vi "Manage Memory.vi"(8 "error in (no error)":errorcluster, 9 "User Waveform (0)":i32, 10 "Memory Operation (0: List Memory)":i32(ring) items=["List Memory", "Copy to User Waveform", "Copy from User Waveform"], 11 "VISA resource name":refnum<visa-resource-name>) -> (0 "error out":errorcluster, 2 "Memory List":string, 3 "VISA resource name out":refnum<visa-resource-name>)   [LabVIEW 2016, in "Tektronix AFG 1000 Series.lvlib"]
doc: "Copy or list memory waveforms."
uses:
  Tektronix AFG 1000 Series.lvlib
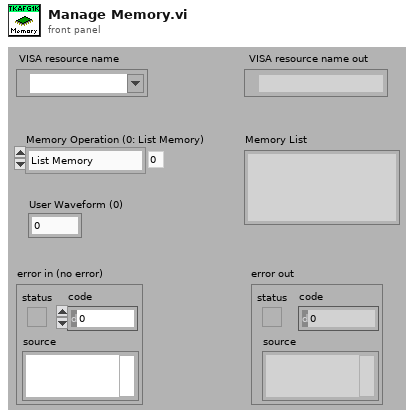
[diagram p1: front panel]
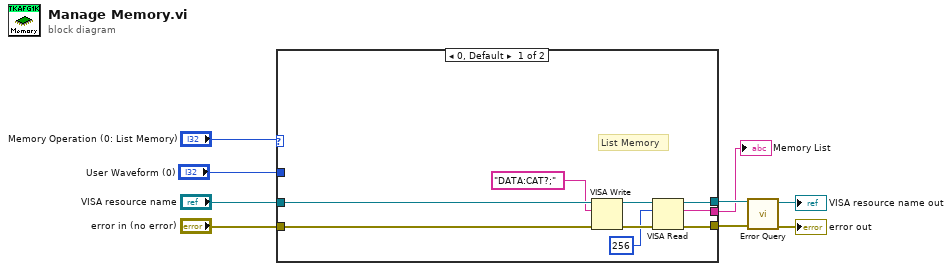
[diagram p0: block diagram]
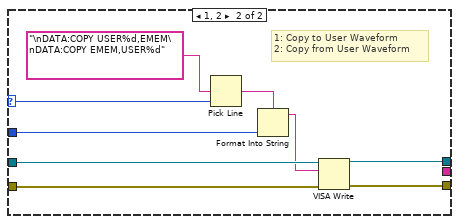
[diagram p2: hidden frame]
diagram:
  n1 = case shown="0, Default" "Memory Operation (0: List Memory)" {
    selector: "Memory Operation (0: List Memory)" -> [_ w27]
    tunnel: "VISA resource name" -> [w18 w25]
    tunnel: "error in (no error)" -> [w17 w24]
    tunnel: [w12 w22] -> w4
    tunnel: [w13 w21] -> w3
    tunnel: [w11 _] -> w2
    tunnel: "User Waveform (0)" -> [_ w19]
    frame 0, Default {
      # "List Memory"
      n2 = VISA Write(VISA resource name=w18, write buffer="DATA:CAT?;" ("string (\"\")"), error in (no error)=w17) -> (VISA resource name out=w15:refnum<visa-resource-name>, error out=w14:errorcluster)  [unwired: 1 out]
      n3 = VISA Read(VISA resource name=w15, byte count=u32 256, error in (no error)=w14) -> (VISA resource name out=w12:refnum<visa-resource-name>, read buffer=w11:string, error out=w13:errorcluster)  [unwired: 1 out]
    }
    frame 1, 2 {
      # "1: Copy to User Waveform\n2: Copy from User Waveform"
      n4 = Pick Line(multi-line string="\nDATA:COPY USER%d,EMEM\nDATA:COPY EMEM,USER%d" ("string (\"\")"), line index=w27) -> (output string=w20:string)  [unwired: 1 in]
      n5 = Format Into String(format string=w20, w19) -> (resulting string=w23:string)  [unwired: 2 in, 1 out]
      n6 = VISA Write(VISA resource name=w25, write buffer=w23, error in (no error)=w24) -> (VISA resource name out=w22:refnum<visa-resource-name>, error out=w21:errorcluster)  [unwired: 1 out]
    }
  }
  "Memory List" <- w2
  n7 = call "Error Query.vi"("error in (no error)"=w3, "VISA resource name"=w4) -> ("error out"=→"error out":errorcluster, "VISA resource name out"=→"VISA resource name out":refnum<visa-resource-name>)  [unwired: 6 in, 2 out]
